vi "Search Yellow Grid.vi"(8 "error in (no error)":errorcluster, 9 "y":sgl, 10 "x":sgl, 11 "Grid for Yellow Player":dbl[][](array[numeric])) -> (0 "error out":errorcluster, 2 "Yellow Player #":i32, 3 "Found in Grid":bool)   [LabVIEW 2015]
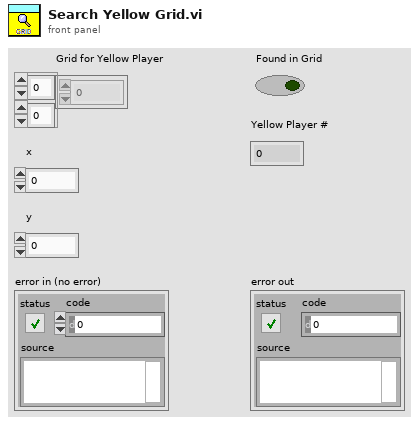
[diagram p1: front panel]
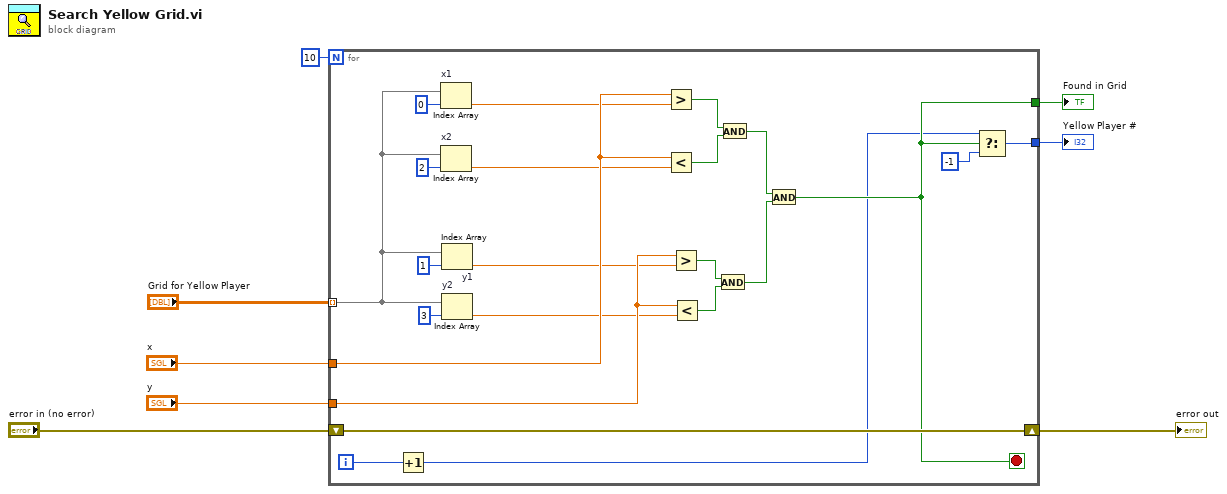
[diagram p0: block diagram]
diagram:
  n1 = for {
    N: 10 -> [_]
    tunnel: "x" -> [w30]
    tunnel: "y" -> [w29]
    shift-right: [w28] -> w3
    shift-left: "error in (no error)" -> [w28]
    tunnel: "Grid for Yellow Player" -> [w23] mode=indexing
    tunnel: [w12] -> w7
    tunnel: [w11] -> w8
    i -> [w31]
    stop <- w11 stop-if-true
    n2 = Increment(x=w31) -> (x+1=w10:i32)
    n3 = Index Array "x1"(array=w23, index=0) -> (element=w22:dbl)
    n4 = Index Array "x2"(array=w23, index=2) -> (element=w20:dbl)
    n5 = Index Array "y1"(array=w23, index=1) -> (element=w21:dbl)
    n6 = Index Array "y2"(array=w23, index=3) -> (element=w19:dbl)
    n7 = Greater?(x=w30, y=w22) -> (0:w13:bool)
    n8 = Less?(x=w30, y=w20) -> (x < y?=w14:bool)
    n9 = Greater?(x=w29, y=w21) -> (0:w16:bool)
    n10 = Less?(x=w29, y=w19) -> (x < y?=w15:bool)
    n11 = And(x=w16, y=w15) -> (x .and. y?=w18:bool)
    n12 = And(x=w13, y=w14) -> (x .and. y?=w17:bool)
    n13 = And(x=w17, y=w18) -> (x .and. y?=w11:bool)
    n14 = Select(t=w10, s=w11, f=-1) -> (s? t:f=w12:i32)
  }
  "Found in Grid" <- w8
  "Yellow Player #" <- w7
  "error out" <- w3
